vi "Create LV RPC Method Name.vi"(1 "Proto Parser RPC Method Name in":string) -> (0 "LV RPC Method Name out":string)   [LabVIEW 2019, in "gRPC Scripting Tools.lvlib"]
uses:
  gRPC Scripting Tools.lvlib
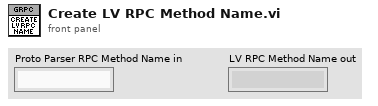
[diagram p1: front panel]
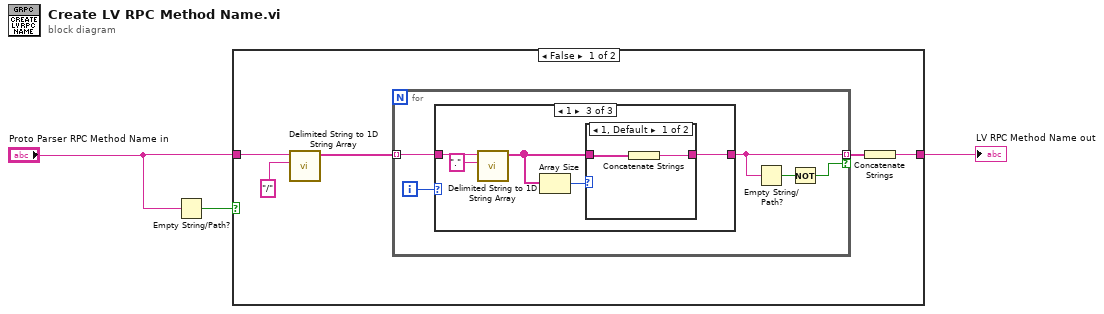
[diagram p0: block diagram]
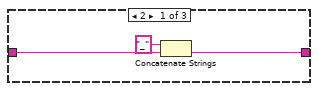
[diagram p2: hidden frame]
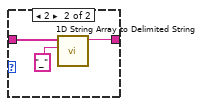
[diagram p4: hidden frame]
diagram:
  n1 = Empty String/Path?(string/path="Proto Parser RPC Method Name in") -> (empty?=w1:bool)
  n2 = case shown="False" w1 {
    tunnel: [w8 w28] -> w3
    tunnel: "Proto Parser RPC Method Name in" -> [w4 w28]
    frame False {
      n3 = call <vilib>:"Delimited String to 1D String Array.vi"("delimiter"="/", "delimited string"=w4) -> ("string array"=w6:string[])  [unwired: 9 in]
      n4 = for {
        tunnel: w6 -> [w12] mode=indexing
        tunnel: [w11] -> w7 mode=indexing if=w9
        i -> [w13]
        n5 = case shown="1" w13 {
          tunnel: w12 -> [w16 w17 w22]
          tunnel: [w15 w17 w20] -> w11
          frame 2 {
            n6 = Concatenate Strings("_" ("string"), w16) -> (w15:string)
          }
          frame 0, Default {
          }
          frame 1 {
            n7 = call <vilib>:"Delimited String to 1D String Array.vi"("delimiter"=".", "delimited string"=w22) -> ("string array"=w19:string[])  [unwired: 9 in]
            n8 = Array Size(array=w19) -> (size(s)=w18:i32)
            n9 = case shown="1, Default" w18 {
              tunnel: [w23 w26] -> w20
              tunnel: w19 -> [w24 w25]
              frame 1, Default {
                n10 = Concatenate Strings(w24) -> (w23:string)
              }
              frame 2 {
                n11 = call <vilib>:"1D String Array to Delimited String.vi"("delimiter"="_", "string array"=w25) -> ("delimited string"=w26:string)  [unwired: 9 in]
              }
            }
          }
        }
        n12 = Empty String/Path?(string/path=w11) -> (empty?=w10:bool)
        n13 = Not(x=w10) -> (.not. x?=w9:bool)
      }
      n14 = Concatenate Strings(w7) -> (w8:string)
    }
    frame True {
    }
  }
  "LV RPC Method Name out" <- w3
